vi "Assign Signal Name and Unit to wForm.vi"(8 "wform IN":waveform(dbl), 11 "Input String":string) -> (0 "wform OUT":waveform(dbl))   [LabVIEW 2020, in "TEXT.lvclass"]
uses:
  TEXT.lvclass
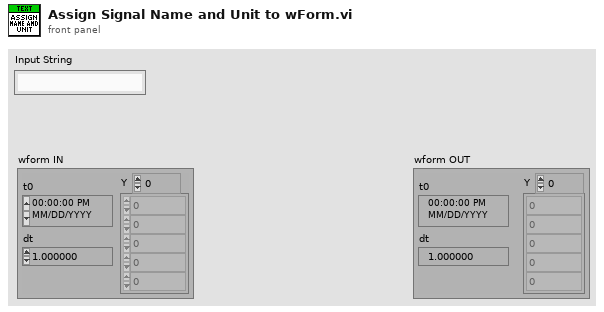
[diagram p1: front panel]
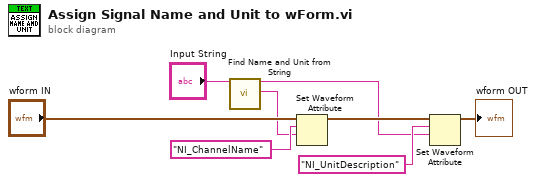
[diagram p0: block diagram]
diagram:
  n1 = call "Find Name and Unit from String.vi"("Input String"="Input String") -> ("Units"=w1:string, "Signal Name"=w2:string)  [unwired: 17 in]
  n2 = Set Waveform Attribute(5:w2, 6:"NI_ChannelName" ("Att - wform Name"), 7:"wform IN") -> (3:w6:waveform(dbl))  [unwired: 1 in, 2 out]
  n3 = Set Waveform Attribute(5:w1, 6:"NI_UnitDescription" ("Att - wform unit"), 7:w6) -> (3:→"wform OUT":waveform(dbl))  [unwired: 1 in, 2 out]
